vi "Read Channel.vi"(8 "error in (no error)":errorcluster, 11 "Initialize_card in":refnum<class "Initialize_card.lvclass">) -> (0 "error out":errorcluster, 2 "Channel":T1={"Coupling"=0, "Differential Input"=FALSE, "Direct-to-ADC"=FALSE, "Range"=2000, "Impedance"=50, "DC Offset"=0, "Filter"=0} {"Impedance" min=50 max=1000000 step=999950; "Coupling" items=["DC", "AC"]}, 3 "Initialize_card out":refnum<class "Initialize_card.lvclass">)   [LabVIEW 2015, in "Initialize_card.lvclass"]
uses:
  Initialize_card.lvclass
  Initialize_card.lvclass/Initialize_card.ctl
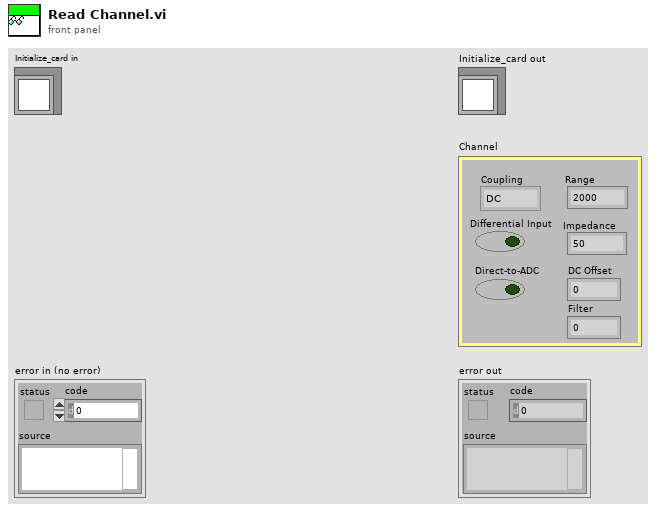
[diagram p1: front panel]
types:
  T1 = cluster{"Coupling":u16, "Differential Input":bool, "Direct-to-ADC":bool, "Range":u32, "Impedance":u32, "DC Offset":i32, "Filter":i32}
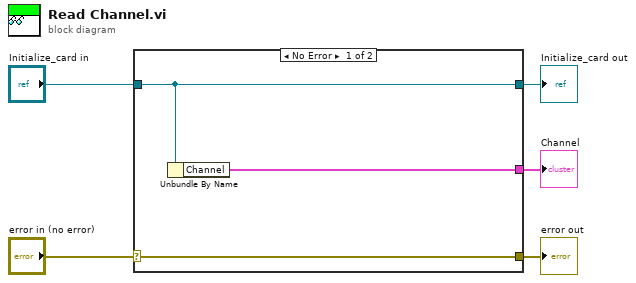
[diagram p0: block diagram]
diagram:
  n1 = case shown="No Error" "error in (no error)" {
    selector: "error in (no error)" -> [w8 w9]
    tunnel: [w8 w9] -> w4
    tunnel: [w7 w10] -> w2
    tunnel: "Initialize_card in" -> [w7 w10]
    tunnel: [w6 _] -> w1
    frame No Error {
      n2 = Unbundle By Name(w7) -> ("Channel"=w6:T1)
    }
    frame Error {
    }
  }
  "error out" <- w4
  "Initialize_card out" <- w2
  "Channel" <- w1
